vi "2_1.vi"() -> ()   [LabVIEW 2015]
panel:
  out "floor(x/y)":dbl
  out "x-y*floor(x/y)":dbl
  out "divide":dbl
  out "multiply":dbl
  out "sub":dbl
  out "sum":dbl
  in  "Y":dbl
  in  "X":dbl
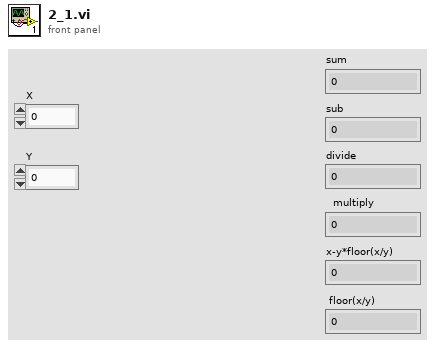
[diagram p1: front panel]
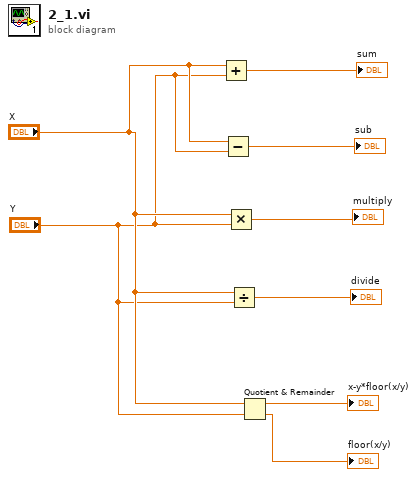
[diagram p0: block diagram]
diagram:
  n1 = Add(x="X", y="Y") -> (x+y=→"sum":dbl)
  n2 = Subtract(x="X", y="Y") -> (x-y=→"sub":dbl)
  n3 = Multiply(x="X", y="Y") -> (x*y=→"multiply":dbl)
  n4 = Divide(x="X", y="Y") -> (x/y=→"divide":dbl)
  n5 = Quotient & Remainder(x="X", y="Y") -> (x-y*floor(x/y)=→"x-y*floor(x/y)":dbl, floor(x/y)=→"floor(x/y)":dbl)
